vi "Alp Led Alloc.vi"(7 "LedId":u32, 8 "error in (no error)":errorcluster, 9 "UserStructPtr":u32, 10 "LedType":i32, 11 "DeviceId":u32) -> (0 "error out":errorcluster, 1 "UserStructPtr out":u32, 3 "function return":i32, 5 "LedId out":u32)   [LabVIEW 2013, in "alpD41.lvlib"]
doc: "ALP_API long ALP_ATTR AlpLedAlloc( ALP_ID DeviceId, long LedType, void *UserStructPtr, ALP_ID *LedId );"
uses:
  <userlib>/alpD41/alpD41.lvlib
  <userlib>/alpD41/alpD41.dll
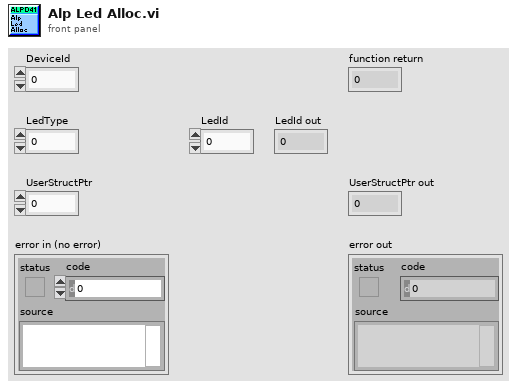
[diagram p1: front panel]
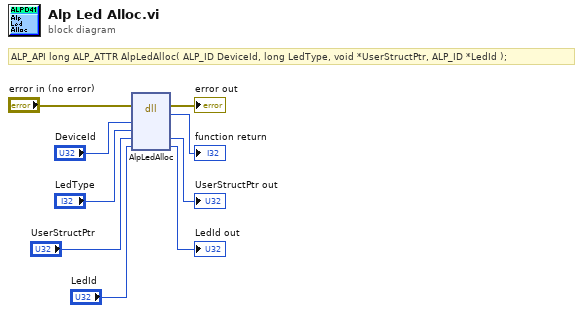
[diagram p0: block diagram]
diagram:
  # "ALP_API long ALP_ATTR AlpLedAlloc( ALP_ID DeviceId, long LedType, void *UserStructPtr, ALP_ID *LedId );"
  n1 = dll-call lib="C:/Program Files (x86)/National Instruments/LabVIEW 2013/user.lib/alpD41/alpD41.*" fn="AlpLedAlloc"(error in="error in (no error)", "DeviceId"="DeviceId", "LedType"="LedType", "UserStructPtr"="UserStructPtr", "LedId"="LedId") -> (error out=→"error out":errorcluster, →"function return":i32, "UserStructPtr"=→"UserStructPtr out":u32, "LedId"=→"LedId out":u32)  [unwired: 4 in, 1 out]
